vi "读标定功率检测值.vi"(11 "VISA资源名称":refnum<visa-resource-name>="COM3") -> (2 "响应":string, 3 "VISA资源名称 2":refnum<visa-resource-name>)   [LabVIEW 2015]
uses:
  E:/National Instruments/LabVIEW 2015/examples/Instrument IO/Serial/support/Serial - Settings.ctl
  <vilib>/Instr/_visa.llb/VISA Configure Serial Port (Instr).vi
panel:
  in  "读取前延时(ms)":u32=500
  in  "串口设置":T1={"波特率"=115200, "数据比特"=8, "奇偶"=enum."None", "停止位"=10, "流控制"=0} {"流控制" items=["无"=0, "XON/XOFF"=1, "RTS/CTS"=2, "DTR/DSR"=4]; "停止位" items=["1.0"=10, "1.5"=15, "2.0"=20]; "数据比特" min=5 max=8 step=1; "波特率" items=["75"=75, "110"=110, "134"=134, "150"=150, "300"=300, "600"=600, "1200"=1200, "1800"=1800, "2400"=2400, "4800"=4800, "7200"=7200, "9600"=9600, "14400"=14400, "19200"=19200, "28800"=28800, "38400"=38400, "56000"=56000, "57600"=57600, "115200"=115200, "128000"=128000, "230400"=230400]}
  out "读取的字节":u32
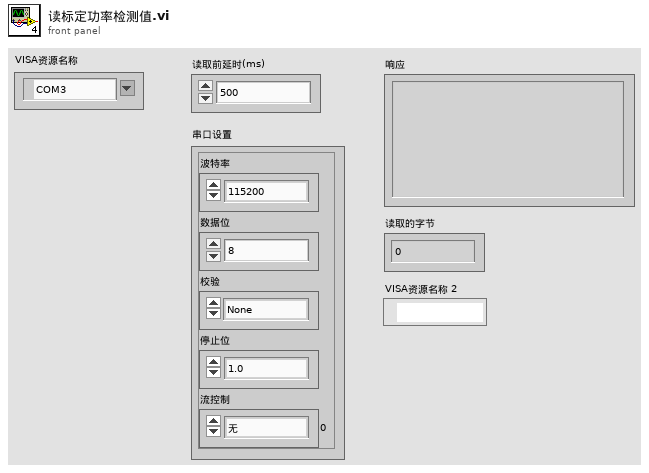
[diagram p1: front panel]
types:
  T1 = typedef "Serial - Settings.ctl" = cluster{"波特率":u32, "数据比特":u16, "奇偶":enum16{"None", "Odd", "Even", "Mark", "Space"}, "停止位":u16, "流控制":u16}
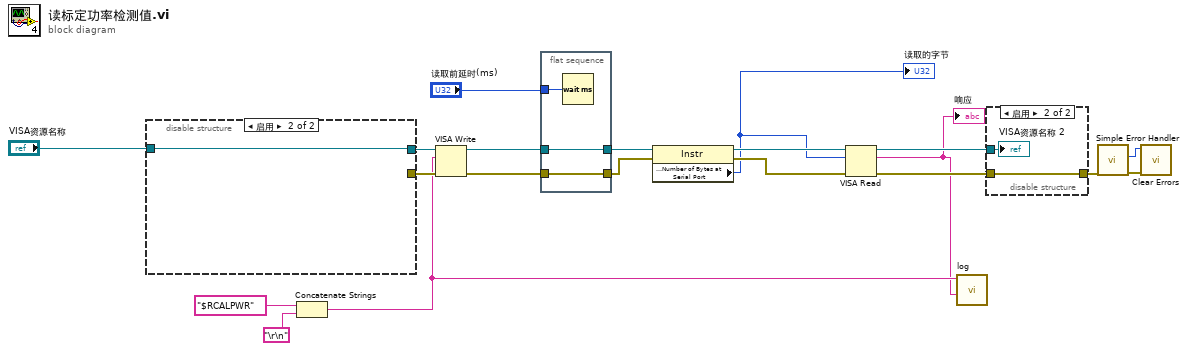
[diagram p0: block diagram]
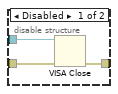
[diagram p2: hidden frame]
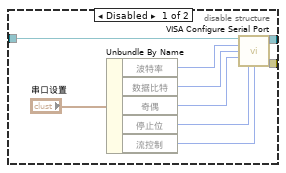
[diagram p3: hidden frame]
diagram:
  n1 = disable-structure shown="启用" {
    disable-tunnel: "VISA资源名称" -> [w29 w30]
    disable-tunnel: [w28 _] -> w19
    disable-tunnel: [w27 w30] -> w18
    frame Disabled {
      n2 = Unbundle By Name("串口设置") -> ("波特率"=w25:u32, "数据比特"=w24:u16, "奇偶"=w23:enum16{"None", "Odd", "Even", "Mark", "Space"}, "停止位"=w22:u16, "流控制"=w21:u16)
      n3 = call-poly "VISA Configure Serial Port"("VISA resource name"=w29, "baud rate (9600)"=w25, "data bits (8)"=w24, "parity (0:none)"=w23, "stop bits (10: 1 bit)"=w22, "flow control (0:none)"=w21) -> ("VISA resource name out"=w27:refnum<visa-resource-name>, "error out"=w28:errorcluster)  [unwired: 3 in, 5 out]
    }
    frame Enabled {
    }
  }
  n4 = Concatenate Strings("$RCALPWR" ("参数"), "\r\n") -> (w2:string)
  n5 = VISA Write(VISA resource name=w18, write buffer=w2, error in (no error)=w19) -> (VISA resource name out=w12:refnum<visa-resource-name>, error out=w11:errorcluster)  [unwired: 1 out]
  n6 = flat-sequence {
    tunnel: w11 -> [w32]
    tunnel: [w32] -> w8
    tunnel: w12 -> [w31]
    tunnel: [w31] -> w9
    tunnel: "读取前延时(ms)" -> [w33]
    frame #0 {
      n7 = Wait (ms)(milliseconds to wait=w33) -> ()  [unwired: 1 out]
    }
  }
  n8 = property class="Instr"(reference=w9, error in=w8) -> (reference out=w7:refnum<visa-resource-name>, error out=w6:errorcluster, "Serial Settings:Number of Bytes at Serial Port"=w5:u32)
  "读取的字节" <- w5
  n9 = VISA Read(VISA resource name=w7, byte count=w5, error in (no error)=w6) -> (VISA resource name out=w16:refnum<visa-resource-name>, read buffer=w1:string, error out=w17:errorcluster)  [unwired: 1 out]
  "响应" <- w1
  n10 = call "log.vi"("响应"=w1, "发送"=w2) -> ()  [unwired: 10 in]
  n11 = disable-structure shown="启用" {
    disable-tunnel: w17 -> [w36 w38]
    disable-tunnel: w16 -> [w35 w37]
    disable-tunnel: [w34 w38] -> w15
    frame Disabled {
      n12 = VISA Close(VISA resource name=w35, error in (no error)=w36) -> (error out=w34:errorcluster)
    }
    frame Enabled {
      "VISA资源名称 2" <- w37
    }
  }
  n13 = call <vilib>:"Simple Error Handler.vi"("error in (no error)"=w15) -> ("code out"=w13:i32, "error out"=w14:errorcluster)  [unwired: 1 in, 6 out]
  n14 = call <vilib>:"Clear Errors.vi"("error in (no error)"=w14, "specific error code to clear (0: all)"=w13) -> ()  [unwired: 4 in, 2 out]
